vi "Load Becker-Hickl File Information String.vi"(8 "Error In":errorcluster, 9 "Info Length":i16, 10 "Info Offset":i32, 11 "File Path in":path) -> (0 "Error Out":errorcluster, 2 "Information String":string, 3 "File Path out":path)   [LabVIEW 2021, in "Becker-Hickl Files.lvlib"]
uses:
  Becker-Hickl Files.lvlib
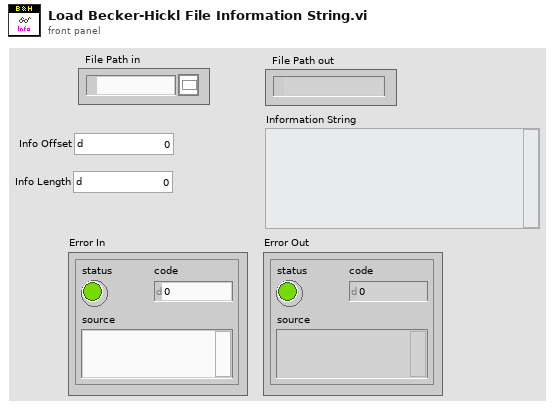
[diagram p1: front panel]
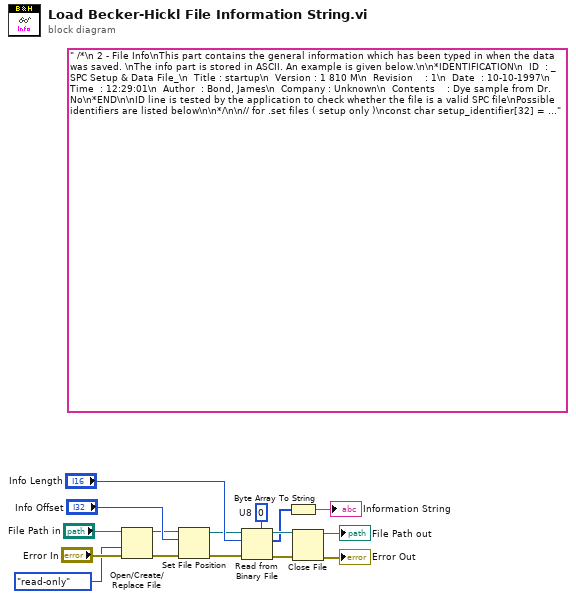
[diagram p0: block diagram]
diagram:
  (unwired) " /*\n 2 - File Info\nThis part contains the general information which has been typed in when the data was saved. \nThe info part is stored in ASCII. An example is given below.\n\n*IDENTIFICATION\n  ID  : _SPC Setup & Data File_\n  Title : startup\n  Version : 1 810 M\n  Revision    : 1\n  Date  : 10-10-1997\n  Time  : 12:29:01\n  Author  : Bond, James\n  Company : Unknown\n  Contents    : Dye sample from Dr. No\n*END\n\nID line is tested by the application to check whether the file is a valid SPC file\nPossible identifiers are listed below\n\n*/\n\n// for .set files ( setup only )\nconst char setup_identifier[32] =      \"\u0004SPC Setup Script File\u0004\"; \n\n// for normal .sdt files ( setup + data )\nconst char  data_identifier[32] =      \"\u0004SPC Setup & Data File\u0004\";\n\n// for .sdt files created automatically in Continuous Flow mode measurement \n//     ( no setup, only data )\nconst char  flow_data_identifier[32] = \"\u0004SPC Flow Data File\u0004\";\n\n// for .sdt files created using DLL function SPC_save_data_to_sdtfile\n//     ( no setup, only data )\nconst char  dll_data_identifier[32]  = \"\u0004SPC DLL Data File\u0004\";\n\n// for .sdt files created in FIFO mode \n//     ( setup, data blocks = Decay, FCS, FIDA, FILDA & MCS curves \n//             for each used routing channel )\nconst char  fcs_data_identifier[32]  = \"\u0004SPC FCS Data File\u0004\";\n"
  w16 = u8 0  # U8
  n1 = Open/Create/Replace File(file path (use dialog)="File Path in", error in="Error In", access (0:read/write)=enum16{"read/write", "read-only", "write-only"}."read-only") -> (refnum out=w11:refnum<file>, error out=w14:errorcluster)  [unwired: 3 in, 1 out]
  n2 = Set File Position(offset (in bytes) (0)="Info Offset", refnum=w11, error in=w14) -> (refnum out=w9:refnum<file>, error out=w8:errorcluster)  [unwired: 1 in]
  n3 = Read from Binary File(5:w16, 8:w8, 10:"Info Length", 11:w9) -> (0:w6:errorcluster, 2:w3:u8[], 3:w7:refnum<file>)  [unwired: 2 in, 1 out]
  n4 = Byte Array To String(unsigned byte array=w3) -> (string=→"Information String":string)
  n5 = Close File(refnum=w7, error in=w6) -> (path=→"File Path out":path, error out=→"Error Out":errorcluster)
